vi "Plink GUI Laser Bay.vi"() -> ()   [LabVIEW 2013]
uses:
  Sandbox/GUI_Template/GUI_master/tcp_new_data_event.ctl
  Sandbox/GUI_Template/GUI_master/tcp new data cluster.ctl
  Non-General/BELLA/VIremote/VIremote.llb/VIremoteFunction.ctl
  <vilib>/Analysis/NI_AALBase.lvlib
panel:
  out "power":dbl=25.5 caption="Power (W)" min=0.0 max=300000000.0 format="%_4p"
  in  "stop":bool
  in  "Clear":bool
  out "XY Graph":cluster{dbl, dbl}[](graph)
  out "sigma":dbl=25.5 caption="Sigma" min=0.0 max=300000000.0 format="%_4p"
  out "mean":dbl=25.5 caption="Mean" min=0.0 max=300000000.0 format="%_4p"
  in  "error IO":errorcluster
  in  "Energy Mode::1":enum16{"off", "on"}(ring) caption="Energy Mode"
  in  "triggerlevel::1":dbl=0.5 caption="Trig Level" min=0.0 max=100.0 format="%_4f"
  out "Wavelength::1":i32 caption="Wavelength" min=0 max=5000
  out "tcp data event":T1
  out "error IO 2":errorcluster
  in  "GUIdevice 1":string="LB_PowerMeter"
  in  "insert tag":bool=TRUE
  in  "Reading::1":dbl=0.5 caption="Power (W)" min=0.0 max=50000.0 format="%_4p"
  # "Laser Bay Power Meter"
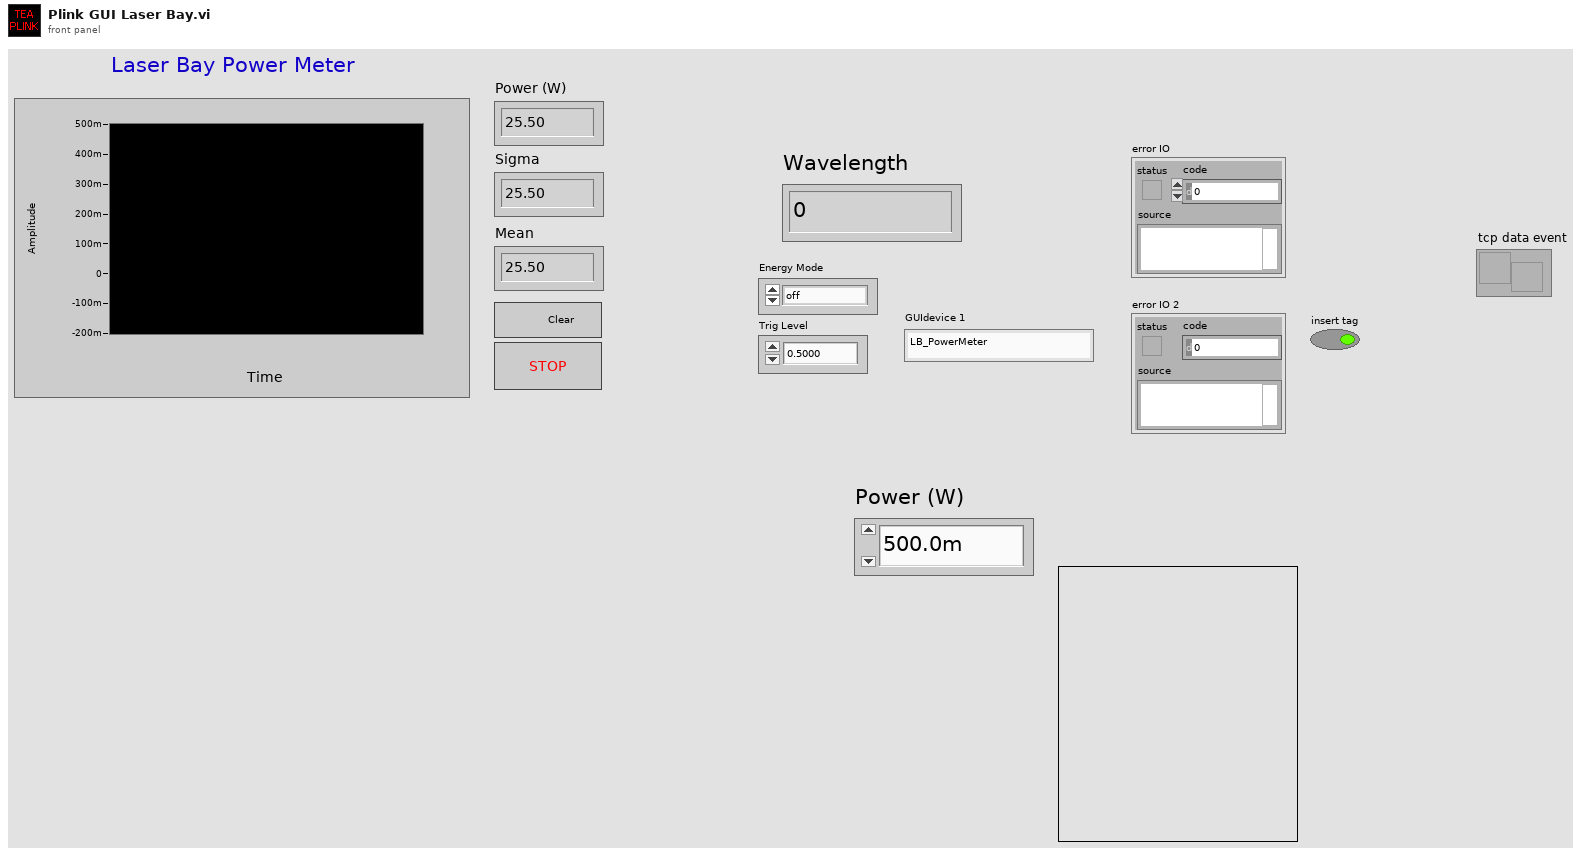
[diagram p1: front panel]
types:
  T1 = typedef "tcp_new_data_event.ctl" = refnum<user-event>
  T2 = typedef "tcp new data cluster.ctl" = cluster{"EventEnum":enum16{"new data", "connection status update"}, "Device name":string}
  T3 = typedef "VIremoteFunction.ctl" = enum16{"Do nothing", "Stop controller", "Close this connection", "Show info panel", "Set VI to control", "Set Accelerometer freq (Hz)", "Show Alert message", "Start Sound Input", "Stop Sound Input", "Set Volume (0-100)", "Set sound output Speaker", "Set sound output Receiver", "Play Sound", "Repeat Sound", "Stop Sound", "Pause Sound", "Resume Sound", "Set panel width of caller (320 or 480)", "Set Panel Size to Portrait", "Set Panel Size to Landscape", "Set Panel Size as Current Orientation", "Allow all UI Orientations", "Send user notification", "Disable Scrolling", "Normal Scrolling", "Page Scrolling", "Set Scroll Offset", "Page Indicator Position"}
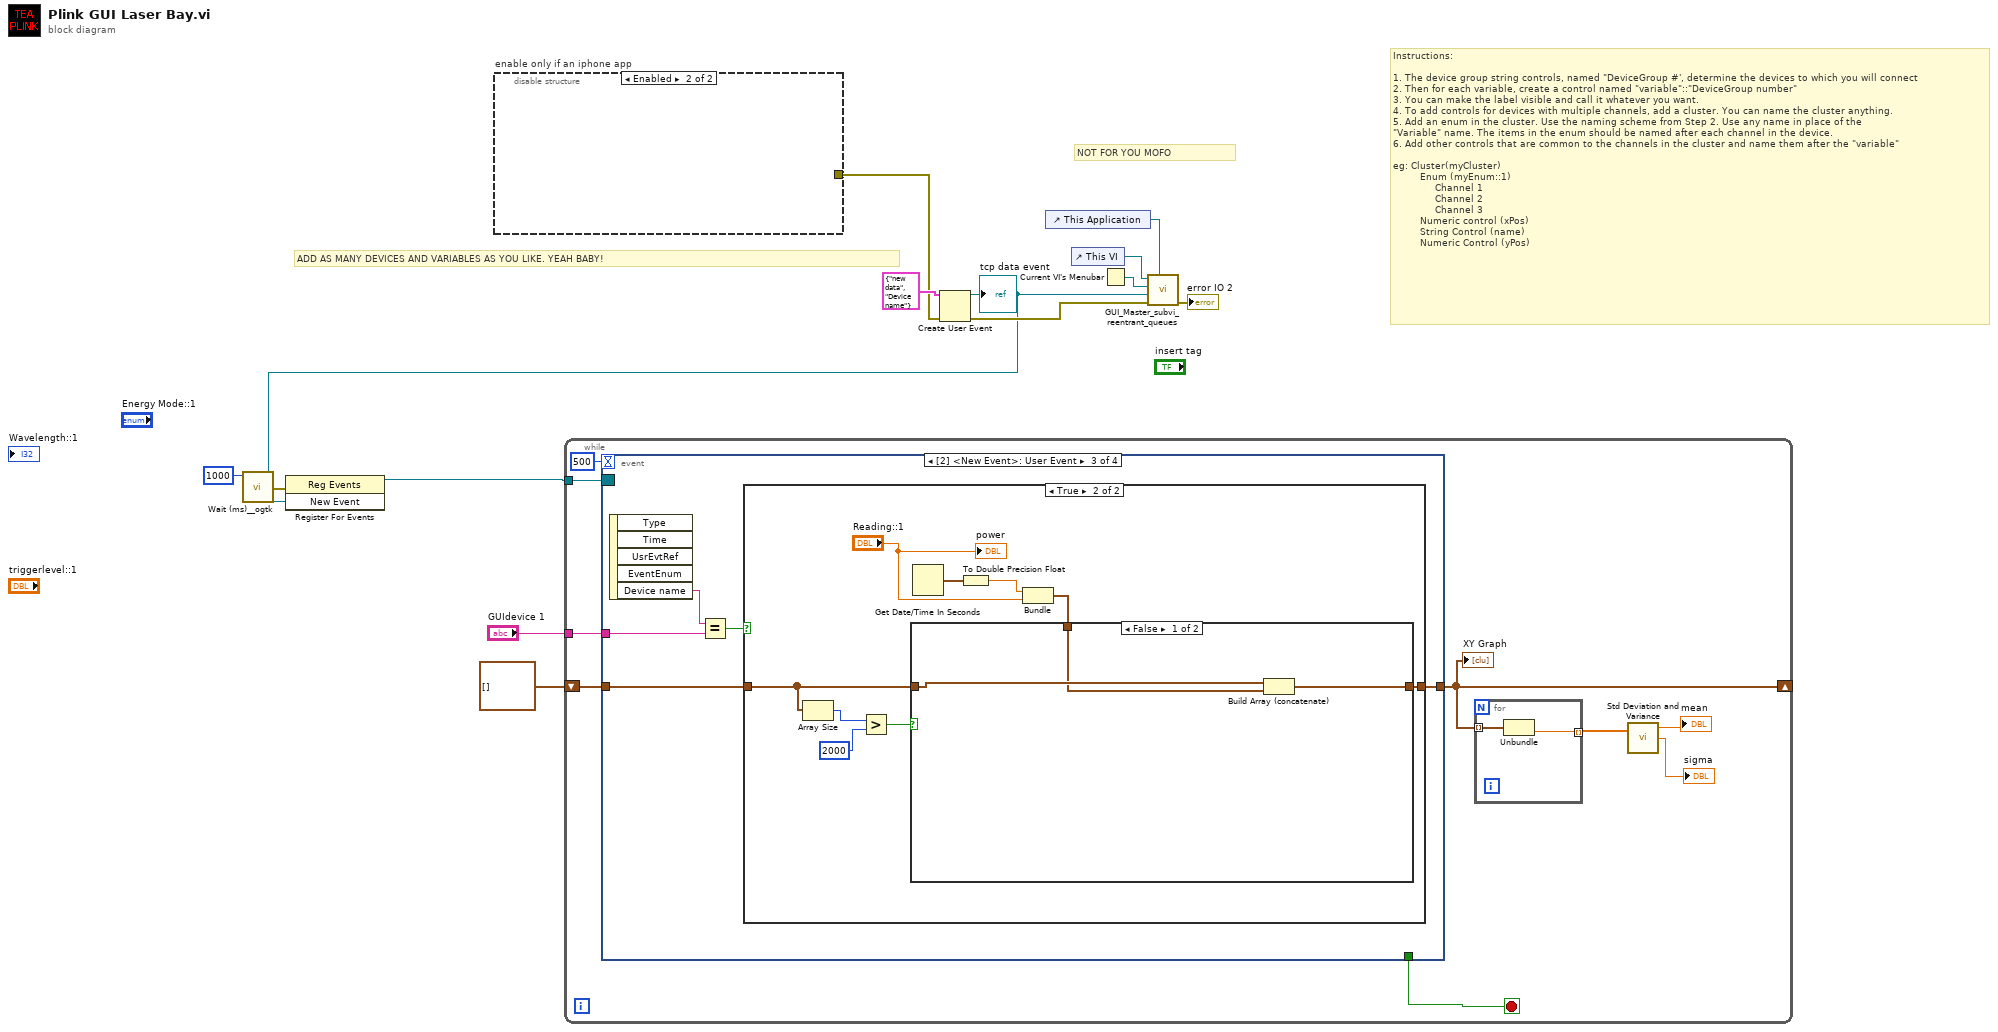
[diagram p0: block diagram]
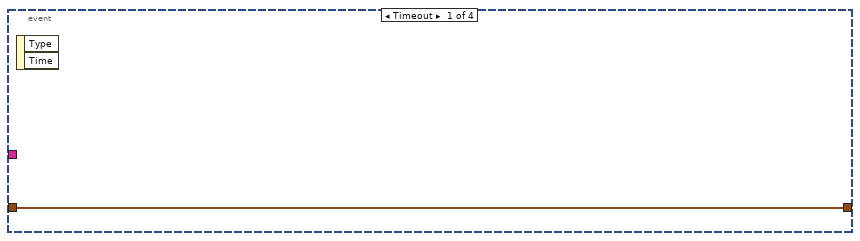
[diagram p2: hidden frame]
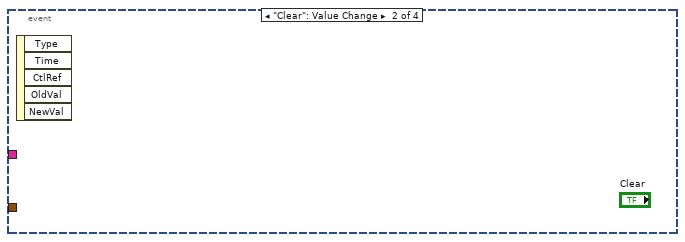
[diagram p3: hidden frame]
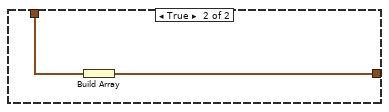
[diagram p5: hidden frame]
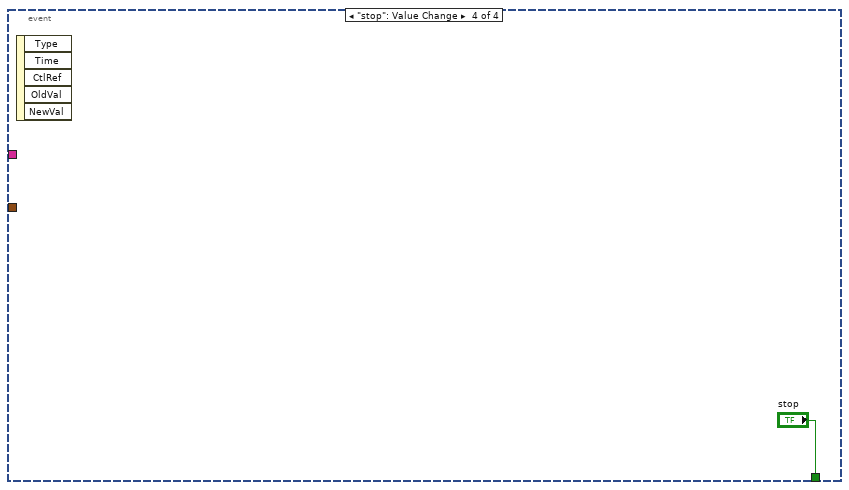
[diagram p6: hidden frame]
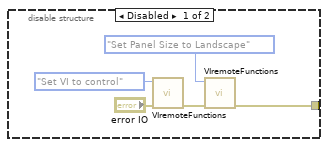
[diagram p7: hidden frame]
diagram:
  # "Instructions:\n\n1. The device group string controls, named \"DeviceGroup #', determine the devices to which you will connect\n2. Then for each variable, create a control named \"variable\"::\"DeviceGroup number\"\n3. You can make the label visible and call it whatever you want.\n4. To add controls for devices with multiple channels, add a cluster. You can name the cluster anything.\n5. Add an enum in the cluster. Use the naming scheme from Step 2. Use any name in place of the \n\"Variable\" name. The items in the enum should be named after each channel in the device. \n6. Add other controls that are common to the channels in the cluster and name them after the \"variable\"\n\neg: Cluster(myCluster)\n         Enum (myEnum::1)\n              Channel 1 \n              Channel 2\n              Channel 3\n         Numeric control (xPos)\n         String Control (name)\n         Numeric Control (yPos)"
  # "ADD AS MANY DEVICES AND VARIABLES AS YOU LIKE. YEAH BABY!"
  # "NOT FOR YOU MOFO"
  n1 = call <userlib>:"Wait (ms)__ogtk.vi"("milliseconds to wait"=u32 1000) -> ("error out"=w1:errorcluster)  [unwired: 9 in, 1 out]
  n2 = disable-structure "enable only if an iphone app" shown="Enabled" {
    disable-tunnel: [w14 _] -> w8
    frame Disabled {
      n3 = call "VIremoteFunctions.vi"("error in (no error)"="error IO", "Function"=VIremoteFunction."Set VI to control") -> ("error out"=w15:errorcluster)  [unwired: 4 in, 5 out]
      n4 = call "VIremoteFunctions.vi"("error in (no error)"=w15, "Function"=VIremoteFunction."Set Panel Size to Landscape") -> ("error out"=w14:errorcluster)  [unwired: 4 in, 5 out]
    }
    frame Enabled {
    }
  }
  n5 = Create User Event(user event datatype=T2 {"EventEnum"=enum."new data", "Device name"="Device name"} ("New Event"), error in=w8) -> (user event=w5:refnum<user-event>, error out=w9:errorcluster)
  "tcp data event" <- w5
  n6 = register-events(error in=w1, w5) -> (reference out=w6:refnum<event-registration>)  [unwired: 1 in, 1 out]
  n7 = while {
    tunnel: w6 -> [w27]
    shift-right: [w23] -> _
    shift-left: cluster{dbl, "data::1":dbl}[] [] -> [w24]
    tunnel: "GUIdevice 1" -> [w19]
    stop <- w25 stop-if-true
    n8 = event shown="[2] <New Event>: User Event" {
      selector: w27 -> [_ _ _ _]
      dyn-events: _ -> [_ _ _ _]
      timeout: 500 -> [_ _ _ _]
      tunnel: [_ _ _ "stop"] -> w25
      tunnel: w24 -> [w30 _ w35 _]
      tunnel: [w30 _ w34 _] -> w23
      tunnel: w19 -> [_ _ w32 _]
      event Timeout {
        n9 = event-data() -> ()  [unwired: 1 in, 2 out]
      }
      event "Clear": Value Change {
        n10 = event-data() -> ()  [unwired: 1 in, 5 out]
      }
      event User Event {
        n11 = event-data() -> ("Device name"=w33:string)  [unwired: 1 in, 4 out]
        n12 = Equal?(x=w33, y=w32) -> (x = y?=w31:bool)
        n13 = case shown="True" w31 {
          tunnel: w35 -> [w36 w45]
          tunnel: [w36 w41] -> w34
          frame False {
          }
          frame True {
            n14 = Array Size(array=w45) -> (size(s)=w44:i32)
            n15 = Greater?(x=w44, y=2000) -> (0:w42:bool)
            n16 = Get Date/Time In Seconds() -> (seconds since 1Jan1904=w39:timestamp)
            n17 = To Double Precision Float(number=w39) -> (double precision float=w40:dbl)
            n18 = Bundle(w40, "Reading::1"="Reading::1") -> (w38:cluster{dbl, "Reading::1":dbl})  [unwired: 1 in]
            n19 = case shown="False" w42 {
              tunnel: w45 -> [w48 _]
              tunnel: [w47 w50] -> w41
              tunnel: w38 -> [w46 w49]
              frame False {
                n20 = Build Array (concatenate)(w48, w46) -> (w47:cluster{dbl, "Reading::1":dbl}[])
              }
              frame True {
                n21 = Build Array(w49) -> (w50:cluster{dbl, "Reading::1":dbl}[])
              }
            }
            "power" <- "Reading::1"
          }
        }
      }
      event "stop": Value Change {
        n22 = event-data() -> ()  [unwired: 1 in, 5 out]
      }
    }
    "XY Graph" <- w23
    n23 = for {
      tunnel: w23 -> [w29] mode=indexing
      tunnel: [w28] -> w22 mode=indexing
      n24 = Unbundle(w29) -> ("Reading::1"=w28:dbl)  [unwired: 1 out]
    }
    n25 = call <vilib>:"Std Deviation and Variance.vi"("X"=w22) -> ("mean"=→"mean":dbl, "standard deviation"=→"sigma":dbl)  [unwired: 1 in, 1 out]
  }
  n26 = control-ref of="This Application"() -> (w2:refnum<vi>)
  n27 = control-ref of="This VI"() -> (w12:refnum<vi>)
  n28 = Current VI's Menubar() -> (w11:refnum<k9>)
  n29 = call "GUI_Master_subvi_reentrant_queues.vi"("This Application"=w2, "error in (no error)"=w9, "tcp data event"=w5, "Caller menu reference"=w11, "Caller VI ref"=w12) -> ("error out"=→"error IO 2":errorcluster)  [unwired: 6 in]
